vi "factorial.vi"(11 "x (input)":u8) -> (3 "x! (output)":u64)   [LabVIEW 2010]
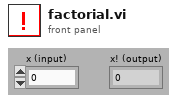
[diagram p1: front panel]
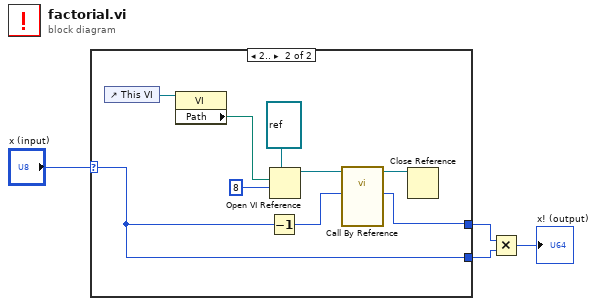
[diagram p0: block diagram]
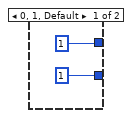
[diagram p2: hidden frame]
diagram:
  n1 = case shown="2.." "x (input)" {
    selector: "x (input)" -> [_ w7]
    tunnel: [u64 1 ("x! (output)") w8] -> w2
    tunnel: [u8 1 ("x (input)") w7] -> w1
    frame 0, 1, Default {
    }
    frame 2.. {
      n2 = control-ref of="This VI"() -> (w15:refnum<vi>)
      n3 = property class="VI"(reference=w15) -> ("Path"=w13:path)  [unwired: 1 in, 2 out]
      n4 = Decrement(x=w7) -> (x-1=w10:u8)
      n5 = Open VI Reference(type specifier VI Refnum (for type only)=refnum<vi> refnum, vi path=w13, options=8) -> (vi reference=w14:refnum<vi>)  [unwired: 3 in, 1 out]
      n6 = call-by-ref "?"(reference=w14, "x (input)"=w10) -> (reference out=w9:refnum<vi>, "x! (output)"=w8:u64)  [unwired: 11 in, 1 out]
      n7 = Close Reference(reference=w9) -> ()  [unwired: 1 in, 1 out]
    }
  }
  n8 = Multiply(x=w2, y=w1) -> (x*y=→"x! (output)":u64)
